vi "Feature Matching.vi"() -> ()   [LabVIEW 2018]
doc: "Feature Matching: This example is the SIFT feature matching example, which establishes correspondence between feature points in different images or between images. These feature points can be prominent local structures in images such as corners, edges, and spots. Find similar features in different images and establish their corresponding relationships for comparison, analysis, or recognition in subsequent image processing tasks."
uses:
  vi.lib/VIRobotics/opencv_yiku/ctls/KeyPoint.ctl
  vi.lib/VIRobotics/opencv_yiku/ctls/Point2f.ctl
  vi.lib/VIRobotics/opencv_yiku/ctls/DMatch.ctl
  vi.lib/VIRobotics/opencv_yiku/Mat/Mat_8U/Mat_8U.lvclass
  D:/Program Files/company/National Instruments/LabVIEW 2018/vi.lib/addons/VIRobotics/opencv_yiku/Mat/Mat/Mat.lvclass
  vi.lib/VIRobotics/opencv_yiku/features2d/vector_KeyPoints/vector_KeyPoint_get_KeyPoints.vi
  vi.lib/VIRobotics/opencv_yiku/features2d/vector_DMatch/get_DMatch.vi
  vi.lib/VIRobotics/opencv_yiku/features2d/vector_DMatch/set_DMatch.vi
  vi.lib/VIRobotics/opencv_yiku/features2d/vector_DMatch/get_size.vi
  vi.lib/VIRobotics/opencv_yiku/features2d/vector_DMatch/vector_DMatch.lvclass
  vi.lib/VIRobotics/opencv_yiku/features2d/vector_KeyPoints/vector_KeyPoint.lvclass
  vi.lib/VIRobotics/opencv_yiku/opencv_yiku.lvlib
  vi.lib/VIRobotics/opencv_yiku/features2d/SIFT/SIFT.lvclass
  vi.lib/VIRobotics/opencv_yiku/features2d/DescriptorMatcher/DescriptorMatcher.lvclass
panel:
  out "size":i32
  out "DMatches":T1[](array[typedef])
  in  "threshold":sgl=0.5
  in  "id":i32
  in  "show all":bool
  out "picture":picture
  out "KeyPoints2":T2[](array[typedef])
  out "KeyPoints1":T2[](array[typedef])
  in  "nfeatures":i32
  out "left":picture
  out "right":picture
  # "Overview: Demonstrates how to match features in one image with others.\nRequirements: Windows.\nInstructions: \n1.Run the VI"
  # "Queryidx corresponds to the array index of the points in KeyPoints1, while trainidx corresponds to the array index of the points in KeyPoints2"
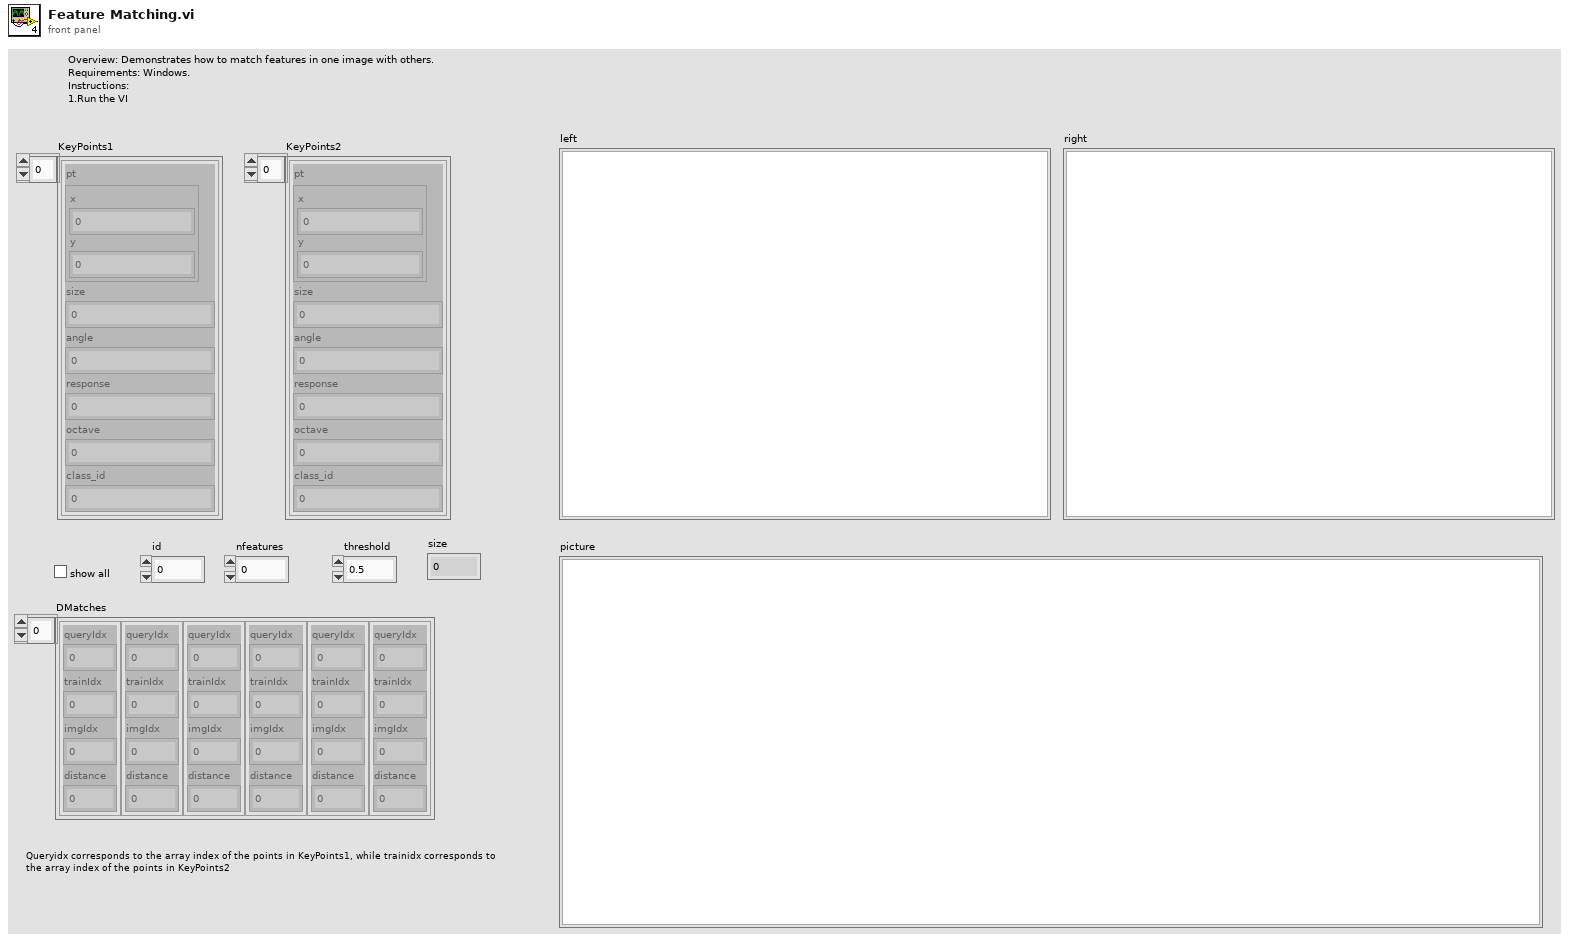
[diagram p1: front panel]
types:
  T1 = typedef "opencv_yiku.lvlib/DMatch.ctl" = cluster{"queryIdx":i32, "trainIdx":i32, "imgIdx":i32, "distance":sgl}
  T2 = typedef "opencv_yiku.lvlib/KeyPoint.ctl" = cluster{"pt":T3, "size":sgl, "angle":sgl, "response":sgl, "octave":i32, "class_id":i32}
  T3 = typedef "opencv_yiku.lvlib/Point2f.ctl" = cluster{"x":sgl, "y":sgl}
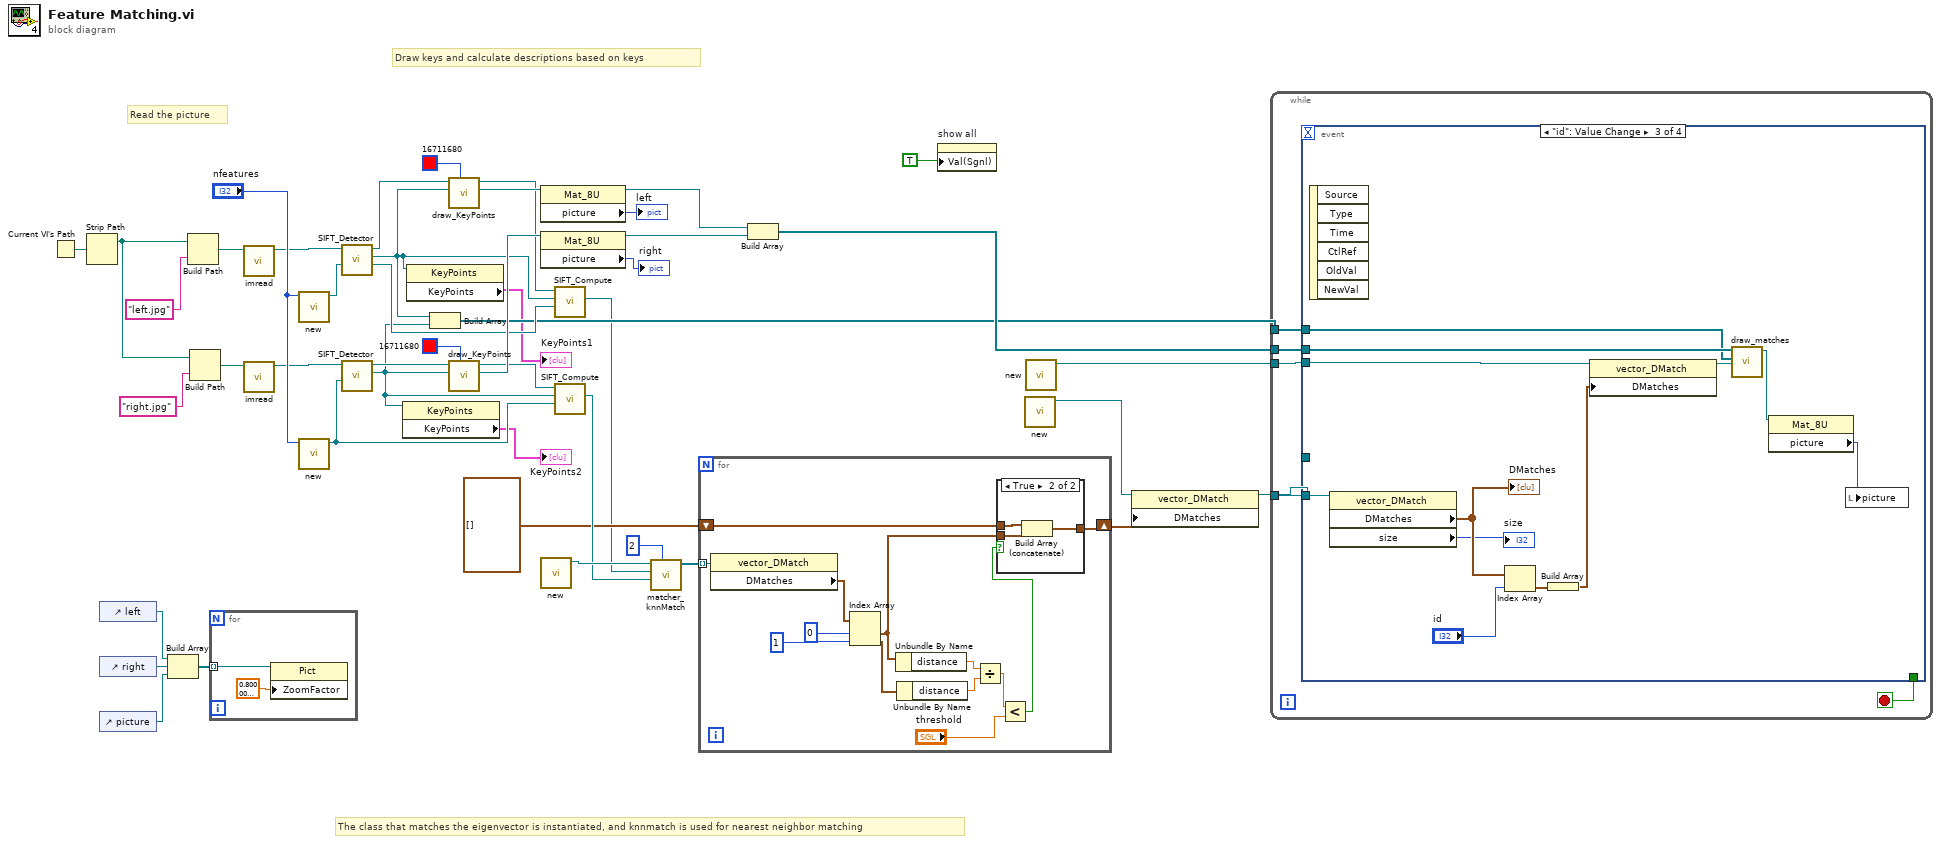
[diagram p0: block diagram]
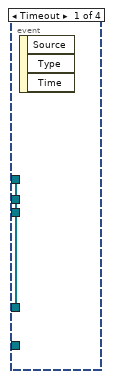
[diagram p3: hidden frame]
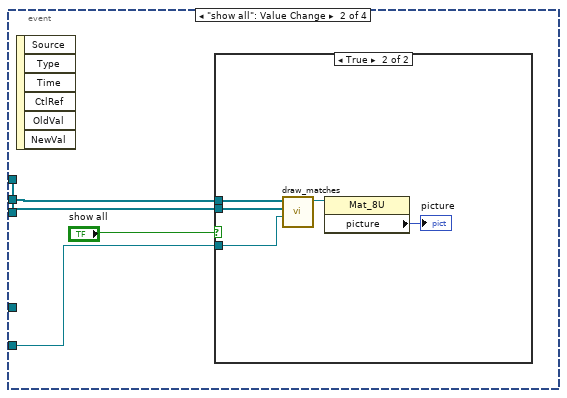
[diagram p4: hidden frame]
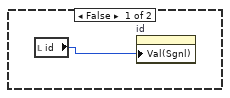
[diagram p5: hidden frame]
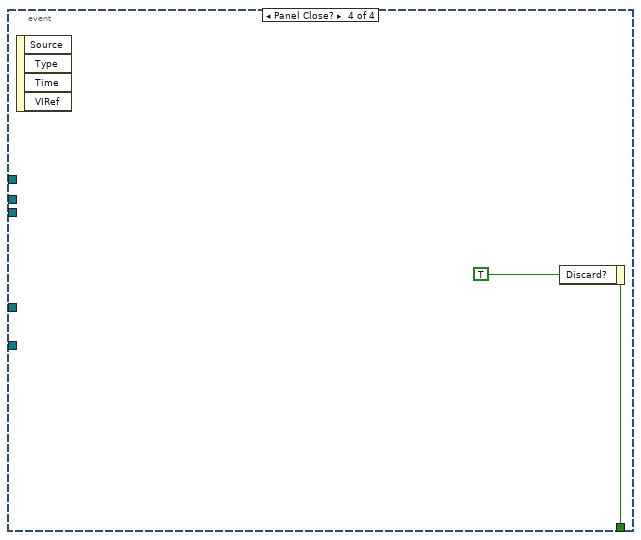
[diagram p6: hidden frame]
diagram:
  # "The class that matches the eigenvector is instantiated, and knnmatch is used for nearest neighbor matching"
  # "Draw keys and calculate descriptions based on keys"
  # "Read the picture"
  n1 = Current VI's Path() -> (path=w15:path)
  n2 = Strip Path(path=w15) -> (stripped path=w11:path)  [unwired: 1 out]
  n3 = control-ref of="left"() -> (w20:refnum<vi>)
  n4 = control-ref of="right"() -> (w19:refnum<vi>)
  n5 = control-ref of="picture"() -> (w18:refnum<vi>)
  n6 = Build Array(w20, w19, w18) -> (w17:refnum<vi>[])
  n7 = Build Path(base path=w11, name or relative path="left.jpg") -> (appended path=w13:path)
  n8 = Build Path(base path=w11, name or relative path="right.jpg") -> (appended path=w10:path)
  n9 = for {
    tunnel: w17 -> [w47] mode=indexing
    n10 = property class="Pict"(reference=w47, "ZoomFactor"=sgl 0.8 ("Zoom Factor")) -> ()  [unwired: 1 in, 2 out]
  }
  n11 = call "imread.vi"("path"=w13) -> ("Mat out"=w22:refnum<class "Mat_8U.lvclass">)  [unwired: 9 in, 1 out]
  n12 = call "imread.vi"("path"=w10) -> ("Mat out"=w21:refnum<class "Mat_8U.lvclass">)  [unwired: 9 in, 1 out]
  n13 = call "new.vi"("nfeatures"="nfeatures") -> ("SIFT out"=w40:refnum<class "SIFT.lvclass">)  [unwired: 9 in, 1 out]
  n14 = call "new.vi"("nfeatures"="nfeatures") -> ("SIFT out"=w28:refnum<class "SIFT.lvclass">)  [unwired: 9 in, 1 out]
  n15 = call "SIFT_Detector.vi"("SIFT"=w40, "img"=w22) -> ("SIFT out"=w27:refnum<class "SIFT.lvclass">, "vector_KeyPoint out"=w2:refnum<class "vector_KeyPoint.lvclass">, "img out"=w37:refnum<class "Mat_8U.lvclass">)  [unwired: 6 in, 1 out]
  n16 = call "SIFT_Detector.vi"("SIFT"=w28, "img"=w21) -> ("vector_KeyPoint out"=w25:refnum<class "vector_KeyPoint.lvclass">, "img out"=w43:refnum<class "Mat_8U.lvclass">)  [unwired: 6 in, 2 out]
  n17 = property class="KeyPoints"(reference=w25) -> ("KeyPoints"=→"KeyPoints2":T2[])  [unwired: 1 in, 2 out]
  n18 = property class="KeyPoints"(reference=w2) -> ("KeyPoints"=→"KeyPoints1":T2[])  [unwired: 1 in, 2 out]
  n19 = Build Array(w2, w25) -> (w23:refnum<class "vector_KeyPoint.lvclass">[])
  n20 = call "draw_KeyPoints.vi"("color"=u32 16711680, "vector_KeyPoint"=w2, "img"=w37) -> ("dst out"=w39:refnum<class "Mat_8U.lvclass">, "img out"=w35:refnum<class "Mat_8U.lvclass">)  [unwired: 6 in, 1 out]
  n21 = call "draw_KeyPoints.vi"("color"=u32 16711680, "vector_KeyPoint"=w25, "img"=w43) -> ("dst out"=w45:refnum<class "Mat_8U.lvclass">, "img out"=w41:refnum<class "Mat_8U.lvclass">)  [unwired: 6 in, 1 out]
  n22 = property class="Mat_8U"(reference=w39) -> (reference out=w34:refnum<class "Mat_8U.lvclass">, "picture"=→"left":picture)  [unwired: 1 in, 1 out]
  n23 = property class="Mat_8U"(reference=w45) -> (reference out=w33:refnum<class "Mat_8U.lvclass">, "picture"=→"right":picture)  [unwired: 1 in, 1 out]
  n24 = call "new.vi"() -> ("DescriptorMatcher out"=w31:refnum<class "DescriptorMatcher.lvclass">)  [unwired: 10 in, 1 out]
  n25 = call "SIFT_Compute.vi"("SIFT"=w27, "vector_KeyPoint"=w2, "img"=w35) -> ("descriptor"=w3:refnum<class "Mat_32F.lvclass">)  [unwired: 6 in, 2 out]
  n26 = call "SIFT_Compute.vi"("SIFT"=w28, "vector_KeyPoint"=w25, "img"=w41) -> ("descriptor"=w30:refnum<class "Mat_32F.lvclass">)  [unwired: 6 in, 2 out]
  n27 = call "matcher_knnMatch.vi"("k"=2, "d2"=w30, "d1"=w3, "matcher"=w31) -> ("Array"=w8:refnum<class "vector_DMatch.lvclass">[])  [unwired: 7 in]
  n28 = for {
    tunnel: w8 -> [w60] mode=indexing
    shift-right: [w49] -> w7
    shift-left: T1[] [] ("DMatches") -> [w51]
    n29 = property class="vector_DMatch"(reference=w60) -> ("DMatches"=w59:T1[])  [unwired: 1 in, 2 out]
    n30 = Index Array(array=w59, index #1=0 ("index"), index #2=1 ("index")) -> (element #1=w50:T1, element #2=w56:T1)
    n31 = Unbundle By Name(w50) -> ("distance"=w55:sgl)
    n32 = Unbundle By Name(w56) -> ("distance"=w54:sgl)
    n33 = Divide(x=w55, y=w54) -> (x/y=w48:sgl)
    n34 = Less?(x=w48, y="threshold") -> (x < y?=w52:bool)
    n35 = case shown="True" w52 {
      tunnel: w51 -> [w61 w64]
      tunnel: w50 -> [_ w63]
      tunnel: [w61 w62] -> w49
      frame False {
      }
      frame True {
        n36 = Build Array (concatenate)(w64, w63) -> (w62:T1[])
      }
    }
  }
  n37 = Build Array(w34, w33) -> (w24:refnum<class "Mat_8U.lvclass">[])
  n38 = property on="show all" class="Bool (strict)"("Val(Sgnl)"=TRUE ("Value (Signaling)")) -> ()  [unwired: 2 in, 2 out]
  n39 = call "new.vi"() -> ("vector_DMatch out"=w5:refnum<class "vector_DMatch.lvclass">)  [unwired: 10 in, 1 out]
  n40 = call "new.vi"() -> ("vector_DMatch out"=w4:refnum<class "vector_DMatch.lvclass">)  [unwired: 10 in, 1 out]
  n41 = property class="vector_DMatch"(reference=w5, "DMatches"=w7) -> (reference out=w6:refnum<class "vector_DMatch.lvclass">)  [unwired: 1 in, 1 out]
  n42 = while {
    tunnel: w6 -> [w69]
    tunnel: w24 -> [w68]
    tunnel: w23 -> [w67]
    tunnel: w4 -> [w65]
    stop <- w66 stop-if-true
    n43 = event shown="[2] \"id\": Value Change" {
      selector: _ -> [_ _ _ _]
      dyn-events: _ -> [_ _ _ _]
      timeout: _ -> [_ _ _ _]
      tunnel: w69 -> [w70 w75 w87 _]
      tunnel: w68 -> [w71 w76 w91 _]
      tunnel: w67 -> [w72 w74 w90 _]
      tunnel: [_ _ _ w95] -> w66
      tunnel: [w72 _ _ _] -> _
      tunnel: [w71 _ _ _] -> _
      tunnel: [w70 _ _ _] -> _
      tunnel: w65 -> [_ _ w88 _]
      event Timeout {
        n44 = event-data() -> ()  [unwired: 1 in, 3 out]
      }
      event "show all": Value Change {
        n45 = event-data() -> ()  [unwired: 1 in, 6 out]
        n46 = case shown="True" "show all" {
          tunnel: w76 -> [_ w80]
          tunnel: w75 -> [_ w78]
          tunnel: w74 -> [_ w79]
          frame False {
            n47 = local read "id"() -> (w77:i32)
            n48 = property on="id" class="DigNum (strict)"("Val(Sgnl)"=w77) -> ()  [unwired: 2 in, 2 out]
          }
          frame True {
            n49 = call "draw_matches.vi"("DMatches"=w78, "kps"=w79, "imgs"=w80) -> ("Mat out"=w82:refnum<class "Mat_8U.lvclass">)  [unwired: 7 in, 1 out]
            n50 = property class="Mat_8U"(reference=w82) -> ("picture"=→"picture":picture)  [unwired: 1 in, 2 out]
          }
        }
      }
      event "id": Value Change {
        n51 = event-data() -> ()  [unwired: 1 in, 6 out]
        n52 = property class="vector_DMatch"(reference=w87) -> ("DMatches"=w86:T1[], "size"=→"size":i32)  [unwired: 1 in, 2 out]
        "DMatches" <- w86
        n53 = Index Array(array=w86, index="id") -> (element=w85:T1)
        n54 = Build Array(w85) -> (w84:T1[])
        n55 = property class="vector_DMatch"(reference=w88, "DMatches"=w84) -> (reference out=w92:refnum<class "vector_DMatch.lvclass">)  [unwired: 1 in, 1 out]
        n56 = call "draw_matches.vi"("DMatches"=w92, "kps"=w90, "imgs"=w91) -> ("Mat out"=w93:refnum<class "Mat_8U.lvclass">)  [unwired: 7 in, 1 out]
        n57 = property class="Mat_8U"(reference=w93) -> ("picture"=w89:picture)  [unwired: 1 in, 2 out]
        n58 = local write "picture"(w89) -> ()
      }
      event Panel Close? {
        w95 = TRUE ("Discard?")
        n59 = event-data() -> ()  [unwired: 1 in, 4 out]
        n60 = event-data("Discard?"=w95) -> ()  [unwired: 1 in, 1 out]
      }
    }
  }
